vi "Send Cmd Write Config.vi"(8 "error in (no error)":errorcluster, 10 "Configuration":T1={"Language"={"Name"=""}, "Path Config"={"Data Folder Path"=path "", "PNG Folder Path"=path "", "mp3 Folder Path"=path ""}, "Image Viewer Config"={"Center Point"={"Size"=3, "Color"=0, "Show?"=FALSE}, "bp Point"={"Size"=3, "Color"=0, "Show?"=FALSE}, "w Point"={"Size"=3, "Color"=0, "Show?"=FALSE}, "b Box"={"Fill Color"=0, "Border Color"=0, "Show?"=FALSE}, "i Box"={"Fill Color"=0, "Border Color"=0, "Show?"=FALSE}, "o Point"={"Size"=3, "Color"=0, "Show?"=FALSE}, "c Point"={"Size"=3, "Color"=0, "Show?"=FALSE}}}, 11 "Configuration Window in":refnum<class "Configuration Window.lvclass">) -> (0 "error out":errorcluster, 3 "Configuration Window out":refnum<class "Configuration Window.lvclass">)   [LabVIEW 2018, in "Configuration Window.lvlib" / "Configuration Window.lvclass"]
uses:
  Configuration Window.lvclass
  C:/Program Files (x86)/National Instruments/LabVIEW 2018/vi.lib/ActorFramework/Actor/Actor.lvclass
  Main Panel/LF2R IDE/Const Configuration.ctl
  Main Panel/LF2R IDE/Const Path Setting.ctl
  Main Panel/LF2R IDE/Const Image Viewer Setting.ctl
  Main Panel/LF2R IDE/LF2R IDE Cmd.ctl
  <vilib>/ActorFramework/Actor/Actor.lvclass/Actor.ctl
  Main Panel/LF2R IDE Messages/LF2R IDE Cmd Msg/LF2R IDE Cmd Msg.lvclass/LF2R IDE Cmd Msg.ctl
  <vilib>/ActorFramework/Message Enqueuer/Message Enqueuer.lvclass/Message Enqueuer.ctl
  <vilib>/ActorFramework/Message Enqueuer/Enqueue.vi
  Main Panel/LF2R IDE Messages/LF2R IDE Cmd Msg/LF2R IDE Cmd Msg.lvclass
  C:/Program Files (x86)/National Instruments/LabVIEW 2018/vi.lib/ActorFramework/Message/Message.lvclass
  <vilib>/ActorFramework/Message Priority Queue/Priority Enqueue.vi
  <vilib>/ActorFramework/Actor/Actor.lvclass
  Main Panel/LF2R IDE/Main Panel.lvclass
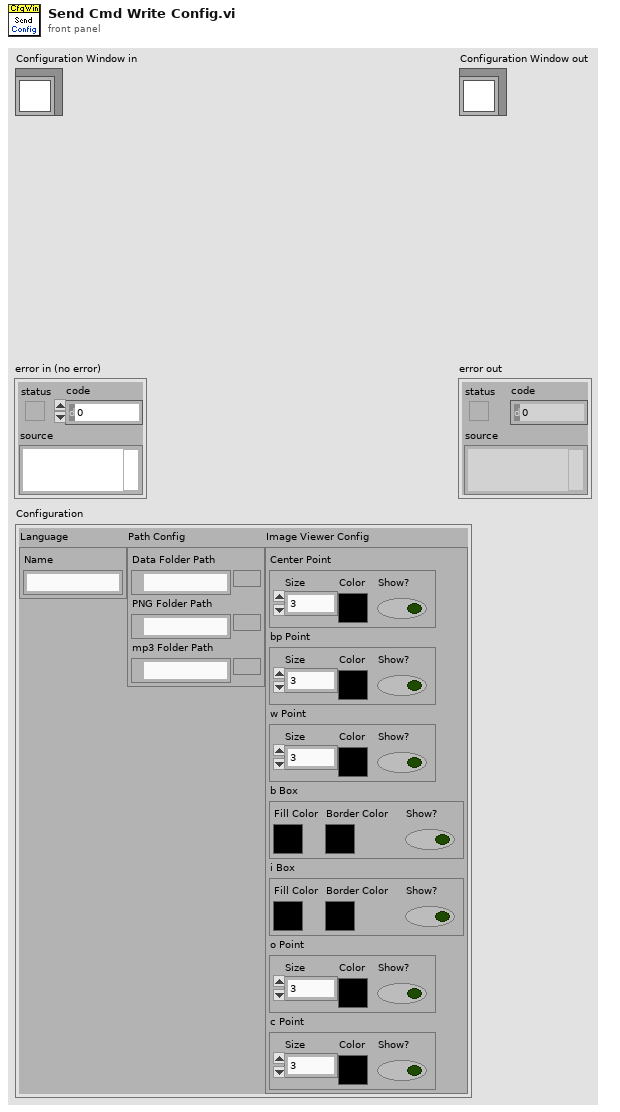
[diagram p1: front panel]
types:
  T1 = typedef "Main Panel.lvlib/Main Panel.lvclass/Const Configuration.ctl" = cluster{"Language":cluster{"Name":string}, "Path Config":T2, "Image Viewer Config":T3}
  T2 = typedef "Main Panel.lvlib/Main Panel.lvclass/Const Path Setting.ctl" = cluster{"Data Folder Path":path, "PNG Folder Path":path, "mp3 Folder Path":path}
  T3 = typedef "Main Panel.lvlib/Main Panel.lvclass/Const Image Viewer Setting.ctl" = cluster{"Center Point":cluster{"Size":i32, "Color":u32, "Show?":bool}, "bp Point":cluster{"Size":i32, "Color":u32, "Show?":bool}, "w Point":cluster{"Size":i32, "Color":u32, "Show?":bool}, "b Box":cluster{"Fill Color":u32, "Border Color":u32, "Show?":bool}, "i Box":cluster{"Fill Color":u32, "Border Color":u32, "Show?":bool}, "o Point":cluster{"Size":i32, "Color":u32, "Show?":bool}, "c Point":cluster{"Size":i32, "Color":u32, "Show?":bool}}
  T4 = typedef "Main Panel.lvlib/Main Panel.lvclass/LF2R IDE Cmd.ctl" = enum16{"Save Data File", "Write Configuration", "Save Configuration", "Update Frame Image"}
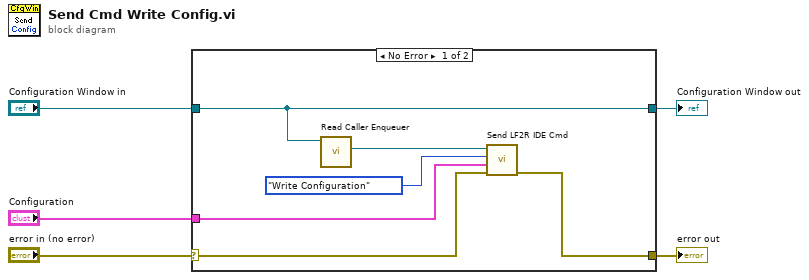
[diagram p0: block diagram]
diagram:
  n1 = case shown="No Error" "error in (no error)" {
    selector: "error in (no error)" -> [w7 w13]
    tunnel: [w6 w13] -> w4
    tunnel: [w11 w12] -> w2
    tunnel: "Configuration Window in" -> [w11 w12]
    tunnel: "Configuration" -> [w8 _]
    frame No Error {
      n2 = call <vilib>:"Read Caller Enqueuer.vi"("Actor"=w11) -> ("Caller Enqueuer"=w10:refnum<class "Message Enqueuer.lvclass">)  [unwired: 10 in]
      n3 = call "Send LF2R IDE Cmd.vi"("error in (no error)"=w7, "Data"=w8, "CMD"=LF2R_IDE_Cmd."Write Configuration", "Message Enqueuer"=w10) -> ("error out"=w6:errorcluster)  [unwired: 6 in, 1 out]
    }
    frame Error {
    }
  }
  "error out" <- w4
  "Configuration Window out" <- w2
